vi "Read 2 measurement Channels Osciloscope.vi"(8 "error in (no error)":errorcluster, 10 "Read 2 channels In":T2={"TEKTRONIX- READ-CHANNELS-IN"={"Channel 1 (1: Channel 1)"=1, "Channel 2 (2: Channel 2)"=2, "Measurement Type (0: Phase)"=0}, "EDU-X-1200A- READ-CHANNELS-IN"={"Timeout (10000 ms)"=10000, "Channels"=[]}} {"EDU-X-1200A- READ-CHANNELS-IN"."Channels" items=["Channel 1"=0, "Channel 2"=1, "Channel 3"=2, "Channel 4"=3, "Waveform Memory 1"=5, "Waveform Memory 2"=6, "Serial Bus 1"=7, "Serial Bus 2"=8, "Digital Bus Low"=9, "Digital Bus High "=10, "Digital Bus 1"=11, "Digital Bus 2"=12, "External"=29, "Function 1"=32, "Function 2"=33, "Function 3"=34, "Function 4"=35, "Math 1"=36, "Math 2"=37, "Math 3"=38, "Math 4"=39, "FFT"=40, "Analog Bus"=41]; "TEKTRONIX- READ-CHANNELS-IN"."Measurement Type (0: Phase)" items=["Phase", "Delay", "DelayRR", "DelayRF", "DelayFR", "DelayFF"]; "TEKTRONIX- READ-CHANNELS-IN"."Channel 2 (2: Channel 2)" items=["Channel 1"=1, "Channel 2"=2, "Channel 3"=3, "Channel 4"=4]; "TEKTRONIX- READ-CHANNELS-IN"."Channel 1 (1: Channel 1)" items=["Channel 1"=1, "Channel 2"=2, "Channel 3"=3, "Channel 4"=4]}, 11 "OsciloscopeClass in":refnum<class "OsciloscopeClass.lvclass">) -> (0 "error out":errorcluster, 2 "Read 2 channels Out":T1, 3 "OsciloscopeClass out":refnum<class "OsciloscopeClass.lvclass">)   [LabVIEW 2020, in "OsciloscopeClass.lvclass"]
uses:
  OsciloscopeClass.lvclass
  TypeDefs/Read2channelsIn--cluster.ctl
  TypeDefs/Read2ChannlesOut.ctl
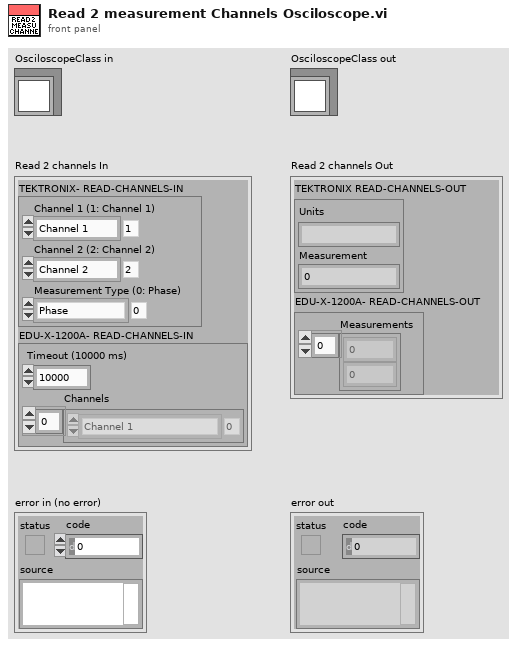
[diagram p1: front panel]
types:
  T1 = typedef "Read2ChannlesOut.ctl" = cluster{"TEKTRONIX READ-CHANNELS-OUT ":cluster{"Units":string, "Measurement":dbl}, "EDU-X-1200A- READ-CHANNELS-OUT":cluster{"Measurements":dbl[]}}
  T2 = typedef "Read2channelsIn--cluster.ctl" = cluster{"TEKTRONIX- READ-CHANNELS-IN":cluster{"Channel 1 (1: Channel 1)":i32, "Channel 2 (2: Channel 2)":i32, "Measurement Type (0: Phase)":i32}, "EDU-X-1200A- READ-CHANNELS-IN":cluster{"Timeout (10000 ms)":u32, "Channels":i32[]}}
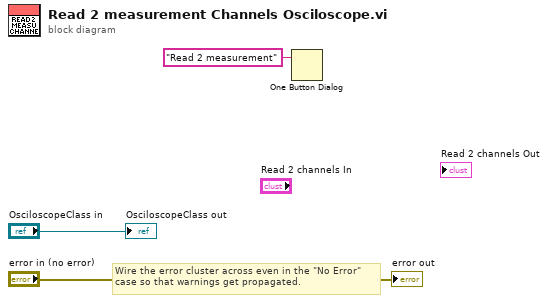
[diagram p0: block diagram]
diagram:
  # "Wire the error cluster across even in the \"No Error\"\ncase so that warnings get propagated."
  n1 = One Button Dialog(message="Read 2 measurement") -> ()  [unwired: 1 in, 1 out]
  "error out" <- "error in (no error)"
  "OsciloscopeClass out" <- "OsciloscopeClass in"
